vi "G_NAV.vi"() -> ()   [LabVIEW 2015]
panel:
  out "GPS_status xxx":T1={"hash"=1114363806672425932, "sys time"=0, "time"=0.0, "x"=0.0, "y"=0.0, "h"=0.0, "numSV"=0, "postype"=0, "lag"=0, "hordev"=0.0, "lat"=0.0, "lon"=0.0, "hgt"=0.0, "map_idx"=0} {"hash" format="%016x"}
  out "M6006_original":T2={"GPSTime"=22892800.0, "accel[0]"=0.0, "accel[1]"=0.0, "accel[2]"=0.0, "pqr[0]"=0.0, "pqr[1]"=0.0, "pqr[2]"=0.0, "llh[0]"=36.366690750000004, "llh[1]"=127.363155, "llh[2]"=72.5, "vel_ned[0]"=0.0, "vel_ned[1]"=0.0, "vel_ned[2]"=0.0, "attitude[0]"=2.0, "attitude[1]"=20.961563, "attitude[2]"=-0.6123908, "vel_bxyz[0]"=0.0, "vel_bxyz[1]"=0.0, "vel_bxyz[2]"=0.0, "lcc[0]"=-970.47205, "lcc[1]"=200.52362, "lcc[2]"=0.0100266, "CovKalman[0]"=0.0, "CovKalman[1]"=0.0, "CovKalman[2]"=0.0, "CovKalman[3]"=0.0, "CovKalman[4]"=0.0, "CovKalman[5]"=0.0, "llh_GPS[0]"=0.0, "llh_GPS[1]"=0.0, "llh_GPS[2]"=0.0, "vel_GPS[0]"=0.0, "vel_GPS[1]"=0.0, "vel_GPS[2]"=0.0, "heading_Magnetic"=0.0, "heading_GPS"=-0.6106907, "GPSStatus"=0, "FailureCode"=0, "DataChecksum"=0} {"GPSTime" format="%#_6f"}
  out "webot ID":refnum<k5>
  in  "ecef ref":dbl[](array[numeric]) format="%#_19f"
  out "NAV Connected?":bool caption="Connection 2"
  out "M2002 header":cluster{u16, u16, u16, u16, u16}={33279, 2002, 12, 36864, 58915}
  out "t7042":string
  out "OEM4POSB_LOG":T3
  out "OEM4_BINARY_HEADER":T4
  out "t6006":string
  out "M60060":T5={"GPSTime"=22892800.0, "attitude[2]"=-0.6123908162117004, "lcc[0]"=-970.4720458984375, "lcc[1]"=200.52362060546875, "heading_GPS"=-0.610690712928772} {"GPSTime" format="%#_6f"}
  out "HEADERWOM":u16[](array[numeric])
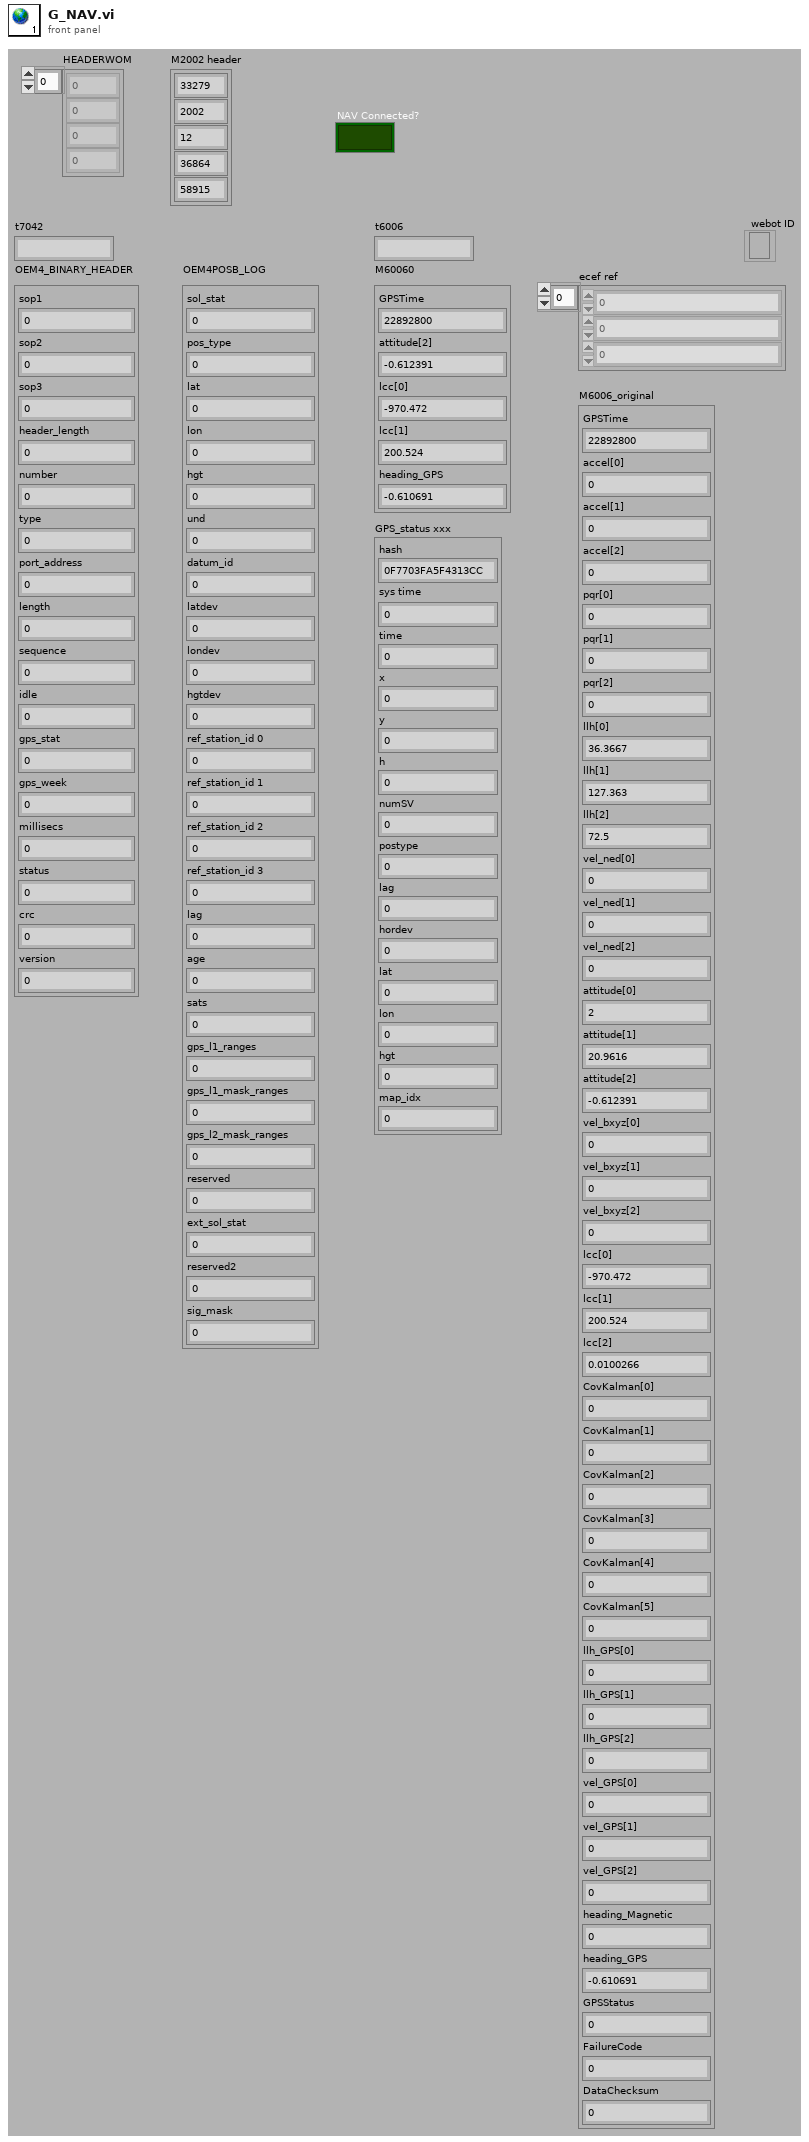
[diagram p1: front panel]
types:
  T1 = cluster{"hash":i64, "sys time":i64, "time":dbl, "x":dbl, "y":dbl, "h":dbl, "numSV":i32, "postype":i32, "lag":i32, "hordev":dbl, "lat":dbl, "lon":dbl, "hgt":dbl, "map_idx":i32}
  T2 = cluster{"GPSTime":dbl, "accel[0]":sgl, "accel[1]":sgl, "accel[2]":sgl, "pqr[0]":sgl, "pqr[1]":sgl, "pqr[2]":sgl, "llh[0]":dbl, "llh[1]":dbl, "llh[2]":dbl, "vel_ned[0]":sgl, "vel_ned[1]":sgl, "vel_ned[2]":sgl, "attitude[0]":sgl, "attitude[1]":sgl, "attitude[2]":sgl, "vel_bxyz[0]":sgl, "vel_bxyz[1]":sgl, "vel_bxyz[2]":sgl, "lcc[0]":sgl, "lcc[1]":sgl, "lcc[2]":sgl, "CovKalman[0]":sgl, "CovKalman[1]":sgl, "CovKalman[2]":sgl, "CovKalman[3]":sgl, "CovKalman[4]":sgl, "CovKalman[5]":sgl, "llh_GPS[0]":sgl, "llh_GPS[1]":sgl, "llh_GPS[2]":sgl, "vel_GPS[0]":sgl, "vel_GPS[1]":sgl, "vel_GPS[2]":sgl, "heading_Magnetic":sgl, "heading_GPS":sgl, "GPSStatus":u16, "FailureCode":u16, "DataChecksum":u16}
  T3 = cluster{"sol_stat":u32, "pos_type":u32, "lat":dbl, "lon":dbl, "hgt":dbl, "und":sgl, "datum_id":i32, "latdev":sgl, "londev":sgl, "hgtdev":sgl, "ref_station_id 0":i8, "ref_station_id 1":i8, "ref_station_id 2":i8, "ref_station_id 3":i8, "lag":sgl, "age":sgl, "sats":u8, "gps_l1_ranges":u8, "gps_l1_mask_ranges":u8, "gps_l2_mask_ranges":u8, "reserved":i8, "ext_sol_stat":u8, "reserved2":u8, "sig_mask":u8}
  T4 = cluster{"sop1":u8, "sop2":u8, "sop3":u8, "header_length":u8, "number":u16, "type":u8, "port_address":u8, "length":u16, "sequence":u16, "idle":u8, "gps_stat":u8, "gps_week":u16, "millisecs":u32, "status":u32, "crc":u16, "version":u16}
  T5 = cluster{"GPSTime":dbl, "attitude[2]":dbl, "lcc[0]":dbl, "lcc[1]":dbl, "heading_GPS":dbl}
diagram:
